vi "UI Message Handler.vi"(8 "error in (no error)":errorcluster) -> (0 "error out":errorcluster)   [LabVIEW 2016]
uses:
  Classes/Lamp/Container/Lamp Container.lvclass
  Controls/Operational Modes.ctl
  Controls/Lamps Manual.ctl
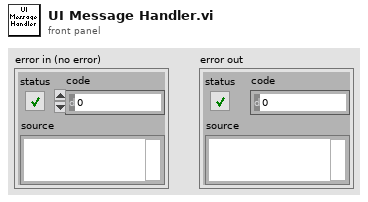
[diagram p1: front panel]
types:
  T1 = typedef "Operational Modes.ctl" = enum16{"Sci", "Sci-LFC", "Solar", "Solar-LFC", "LFC", "LFC-Sim", "LFC-Both", "ThAr", "ThAr-LFC", "Flat", "ExtFlat", "ExtFlat-Sim", "ExtFlat-Both", "Qtz", "ExtQtz", "ExtQtz-Sim", "ExtQtz-Both", "Dark", "Manual", "Off"}
  T2 = typedef "Lamps Manual.ctl" = cluster{"ThAr":bool, "Quartz":bool, "LED":bool, "ThAr Timeout":dbl, "LED Timeout":dbl, "Quartz Timeout":dbl}
  T3 = typedef "Lamps.ctl" = cluster{"ThAr":cluster{"Time Stamp":timestamp, "Status":bool, "Timeout":dbl}, "LED":cluster{"Time Stamp":timestamp, "Status":bool, "Timeout":dbl}, "Quartz":cluster{"Time Stamp":timestamp, "Status":bool, "Timeout":dbl}}
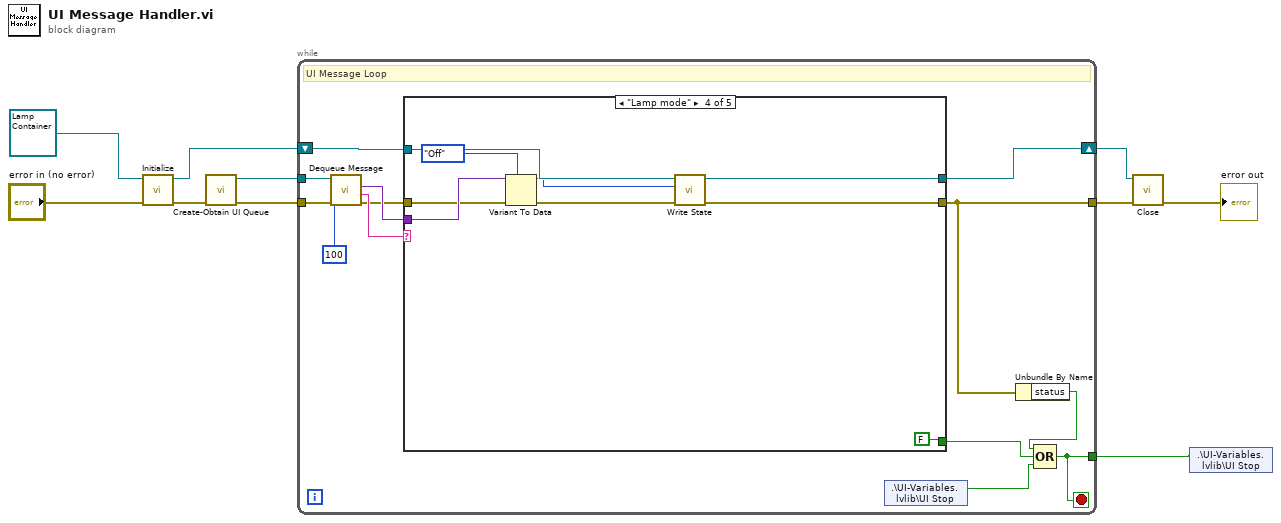
[diagram p0: block diagram]
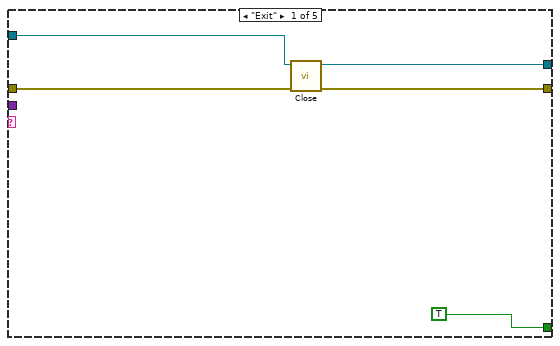
[diagram p2: hidden frame]
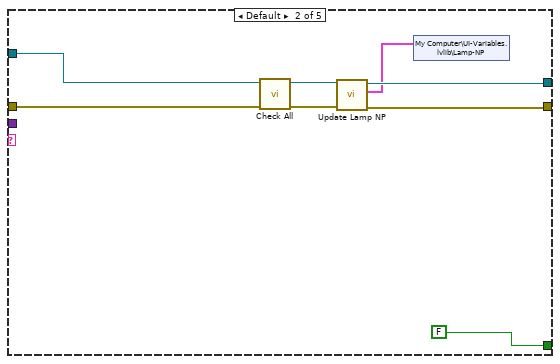
[diagram p3: hidden frame]
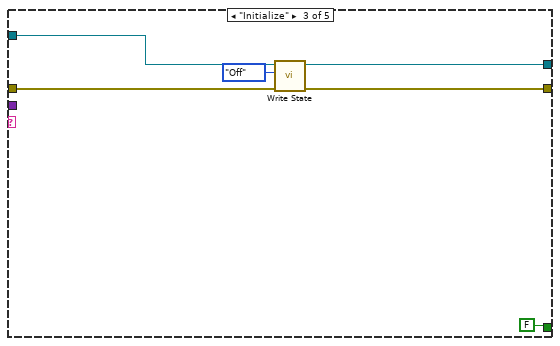
[diagram p4: hidden frame]
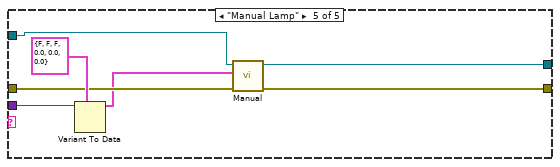
[diagram p5: hidden frame]
diagram:
  n1 = call-dynamic "Initialize.vi"("error in (no error)"="error in (no error)", "Lamp Container in"=refnum<class "Lamp Container.lvclass"> refnum ("Lamp Container.lvclass")) -> ("error out"=w2:errorcluster, "Lamp Container out"=w7:refnum<class "Lamp Container.lvclass">)  [unwired: 8 in]
  n2 = call "Create-Obtain UI Queue.vi"("error in (no error)"=w2) -> ("error out"=w1:errorcluster, "Queue out"=w3:refnum<queue>)  [unwired: 9 in]
  n3 = while {
    tunnel: w3 -> [w17]
    tunnel: [w19] -> w6
    tunnel: w1 -> [w18]
    tunnel: [w21] -> w10
    shift-right: [w11] -> w4
    shift-left: w7 -> [w12]
    stop <- w21 stop-if-true
    # "UI Message Loop"
    n4 = call "Dequeue Message.vi"("error in (no error)"=w18, "timeout in ms (-1)"=100, "Queue in"=w17) -> ("error out"=w14:errorcluster, "Cmd"=w16:string, "Data"=w15:variant)  [unwired: 5 in, 1 out]
    n5 = case shown="\"Lamp mode\"" w16 {
      tunnel: [TRUE FALSE FALSE FALSE _] -> w23
      tunnel: w15 -> [_ _ _ w51 w58]
      tunnel: w14 -> [w27 w34 w40 w49 w54]
      tunnel: [w26 w32 w39 w45 w55] -> w19
      tunnel: w12 -> [w24 w35 w42 w48 w53]
      tunnel: [w25 w31 w38 w47 w56] -> w11
      frame "Exit" {
        n6 = call-dynamic "Close.vi"("error in (no error)"=w27, "Lamp Container in"=w24) -> ("error out"=w26:errorcluster, "Lamp Container out"=w25:refnum<class "Lamp Container.lvclass">)  [unwired: 8 in]
      }
      frame Default {
        n7 = call-dynamic "Check All.vi"("error in (no error)"=w34, "Lamp Container in"=w35) -> ("error out"=w33:errorcluster, "Lamp Container out"=w30:refnum<class "Lamp Container.lvclass">)  [unwired: 8 in]
        n8 = call "Update Lamp NP.vi"("error in (no error)"=w33, "Lamp Container In"=w30) -> ("error out"=w32:errorcluster, "Lamps"=w29:T3, "Lamp Container Out"=w31:refnum<class "Lamp Container.lvclass">)  [unwired: 7 in]
        n9 = shared-variable "My Computer\\UI-Variables.lvlib\\Lamp-NP"(w29) -> ()  [unwired: 1 in, 1 out]
      }
      frame "Initialize" {
        n10 = call-dynamic "Write State.vi"("error in (no error)"=w40, "OpMode"=Operational_Modes."Off", "Lamp Container in"=w42) -> ("error out"=w39:errorcluster, "Lamp Container out"=w38:refnum<class "Lamp Container.lvclass">)  [unwired: 7 in]
      }
      frame "Lamp mode" {
        n11 = Variant To Data(error in=w49, type=Operational_Modes."Off" ("EXPRES Mode 2"), Variant=w51) -> (data=w44:T1, error out=w46:errorcluster)
        n12 = call-dynamic "Write State.vi"("error in (no error)"=w46, "OpMode"=w44, "Lamp Container in"=w48) -> ("error out"=w45:errorcluster, "Lamp Container out"=w47:refnum<class "Lamp Container.lvclass">)  [unwired: 7 in]
      }
      frame "Manual Lamp" {
        n13 = Variant To Data(type=T2 {"ThAr"=FALSE, "Quartz"=FALSE, "LED"=FALSE, "ThAr Timeout"=0.0, "LED Timeout"=0.0, "Quartz Timeout"=0.0} ("Manual Lamp"), Variant=w58) -> (data=w52:T2)  [unwired: 1 in, 1 out]
        n14 = call-dynamic "Manual.vi"("error in (no error)"=w54, "Manual Lamp"=w52, "Lamp Container in"=w53) -> ("error out"=w55:errorcluster, "Lamp Container out"=w56:refnum<class "Lamp Container.lvclass">)  [unwired: 7 in]
      }
    }
    n15 = shared-variable ".\\UI-Variables.lvlib\\UI Stop"() -> (w22:bool)  [unwired: 1 in, 1 out]
    n16 = Unbundle By Name(w19) -> ("status"=w20:bool)
    n17 = Compound Arithmetic op=OR(w20, w23, w22) -> (w21:bool)
  }
  n18 = call-dynamic "Close.vi"("error in (no error)"=w6, "Lamp Container in"=w4) -> ("error out"=→"error out":errorcluster)  [unwired: 8 in, 1 out]
  n19 = shared-variable ".\\UI-Variables.lvlib\\UI Stop"(w10) -> ()  [unwired: 1 in, 1 out]
